vi "write_first_line_and_header.vi"(2 "first_line":string, 3 "Path":path) -> (0 "error out":errorcluster, 1 "Byte Stream File out":refnum<file>)   [LabVIEW 2013]
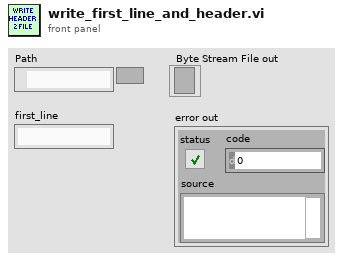
[diagram p1: front panel]
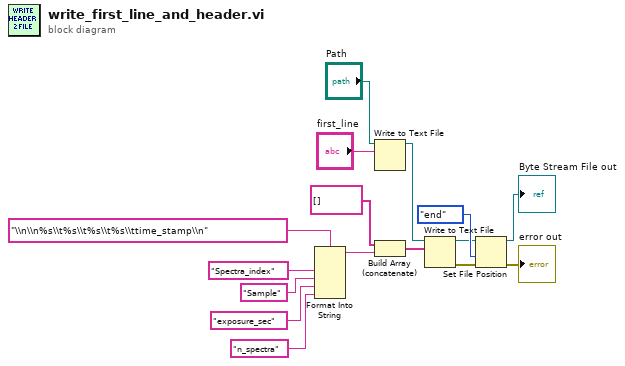
[diagram p0: block diagram]
diagram:
  n1 = Format Into String(format string="\\n\\n%s\\t%s\\t%s\\t%s\\ttime_stamp\\n", "Spectra_index" ("Header 1"), "Sample" ("Header 2"), "exposure_sec" ("Header 3"), "n_spectra" ("Header 4")) -> (resulting string=w5:string)  [unwired: 2 in, 1 out]
  n2 = Write to Text File(file (use dialog)="Path", text="first_line") -> (refnum out=w13:refnum<file>)  [unwired: 2 in, 2 out]
  n3 = Build Array (concatenate)(string[] [], w5) -> (w6:string[])
  n4 = Write to Text File(file (use dialog)=w13, text=w6) -> (refnum out=w7:refnum<file>, error out=w8:errorcluster)  [unwired: 2 in, 1 out]
  n5 = Set File Position(refnum=w7, from (0:start)=enum16{"start", "end", "current"}."end", error in=w8) -> (refnum out=→"Byte Stream File out":refnum<file>, error out=→"error out":errorcluster)  [unwired: 1 in]
